vi "Control - Generic - Fuel Cut Host.vi"() -> ()   [LabVIEW 2015, in "ECS-Host.lvlib"]
uses:
  ECS-Host.lvlib
panel:
  in  "ReengageSpeed":sgl caption="[]"
  in  "MaxEngineSpeed":sgl caption="[]"
  in  "OverspeedFuelQty":sgl caption="[mg/cyc]"
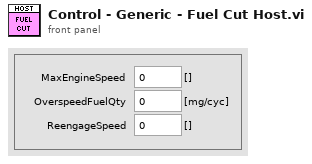
[diagram p1: front panel]
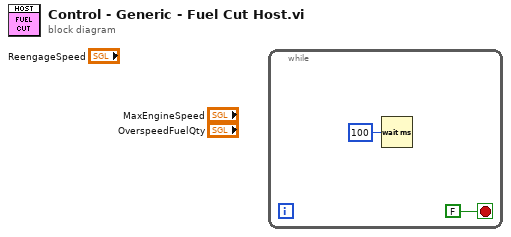
[diagram p0: block diagram]
diagram:
  n1 = while {
    stop <- FALSE stop-if-true
    n2 = Wait (ms)(milliseconds to wait=u32 100) -> ()  [unwired: 1 out]
  }
